vi "IO Channel Configuration.vi"() -> ()   [LabVIEW 2013]
panel:
  out "Sum Input Channel":string
  out "Division Input Channel":string
  out "Y Input Channel":string
  out "X Output Channnel":string
  out "X Input Channel":string
  out "Y Output Channel":string
  out "Z Output Channel":string
  out "Z Input Channel":string
  in  "OK Button":bool
  in  "Enable Y Output":bool=TRUE
  in  "Enable Y Input":bool=TRUE
  in  "Enable X Output":bool=TRUE
  in  "Enable X Input":bool=TRUE
  in  "Division Input Channel":tag
  in  "Sum Input Channel":tag
  in  "Z Output Channel":tag
  in  "Z Input Channel":tag
  in  "Y Output Channel":tag
  in  "Y Input Channel":tag
  in  "X Output Channel":tag
  in  "X Input Channel":tag
  # "Current Values:"
  # "Input/Ouput DAQmx Channel Selection:"
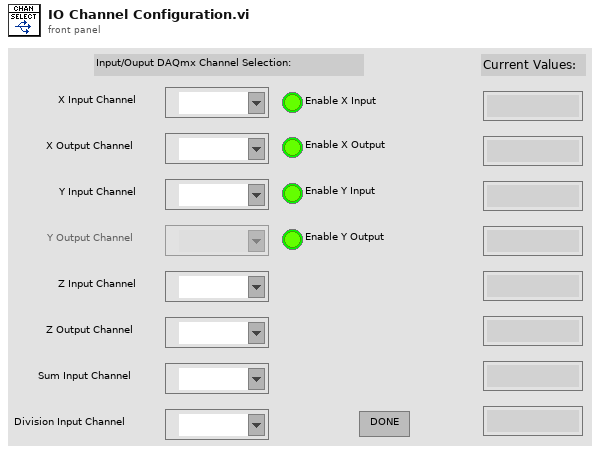
[diagram p1: front panel]
types:
  T1 = enum8{"Enabled", "Disabled", "Disabled and Grayed Out"}
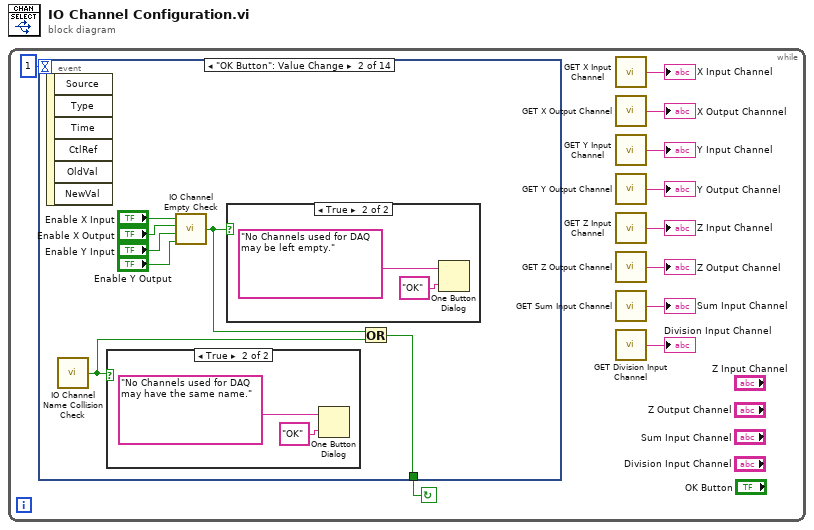
[diagram p0: block diagram]
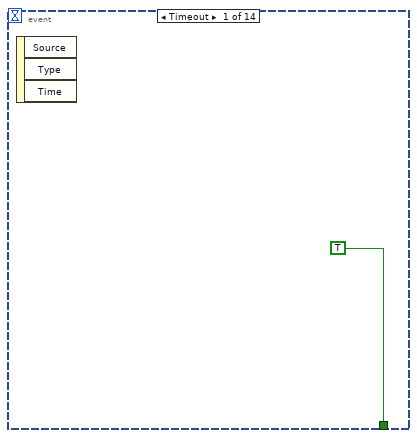
[diagram p2: hidden frame]
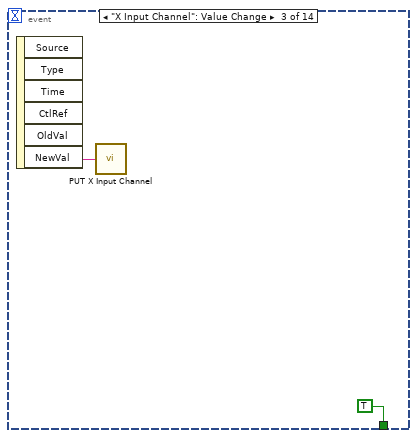
[diagram p5: hidden frame]
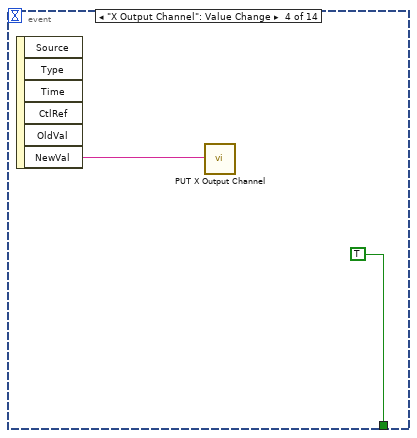
[diagram p6: hidden frame]
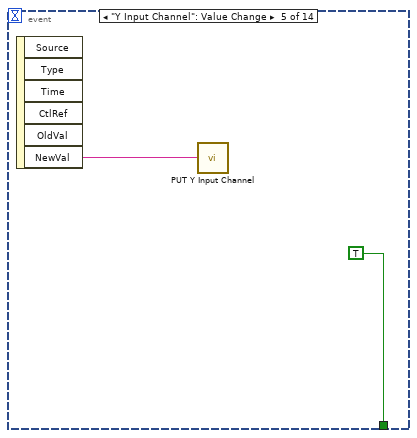
[diagram p7: hidden frame]
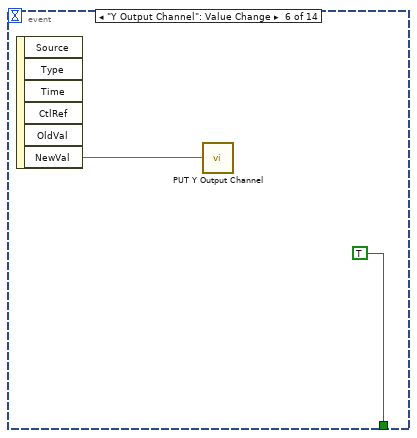
[diagram p8: hidden frame]
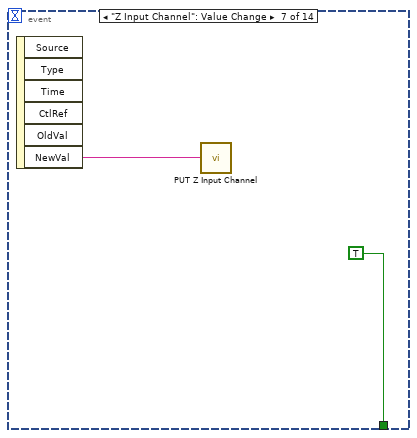
[diagram p9: hidden frame]
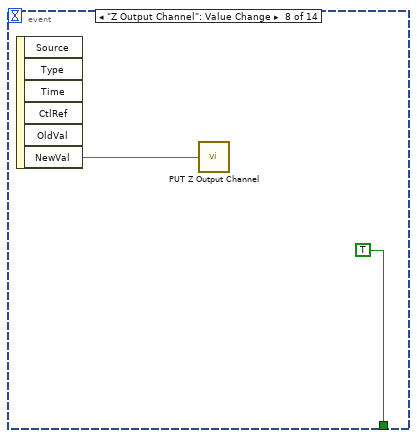
[diagram p10: hidden frame]
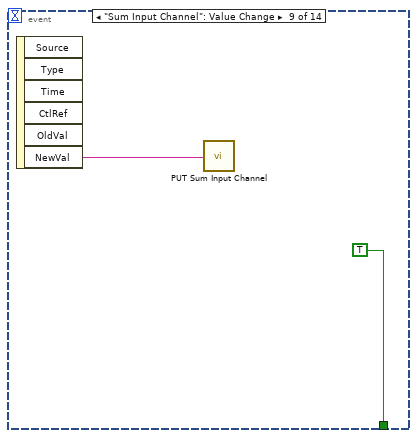
[diagram p11: hidden frame]
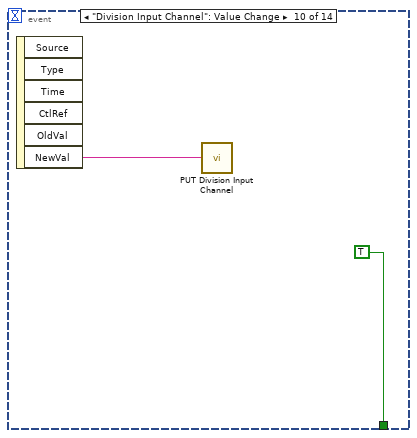
[diagram p12: hidden frame]
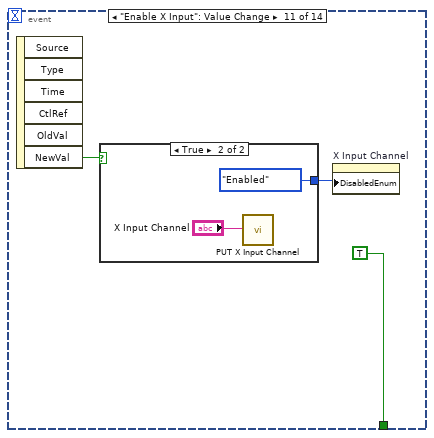
[diagram p13: hidden frame]
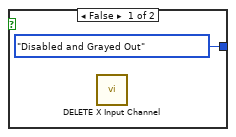
[diagram p14: hidden frame]
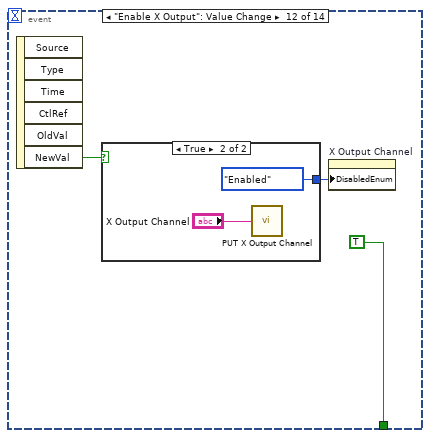
[diagram p15: hidden frame]
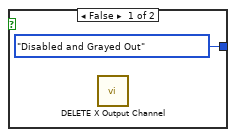
[diagram p16: hidden frame]
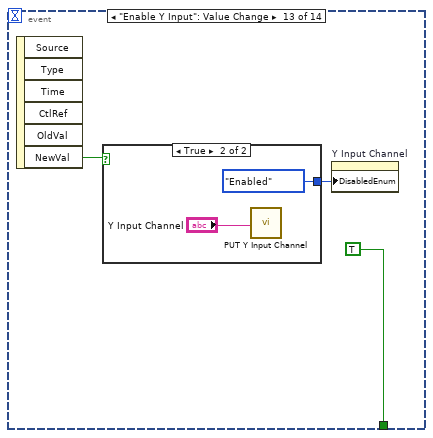
[diagram p17: hidden frame]
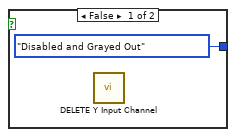
[diagram p18: hidden frame]
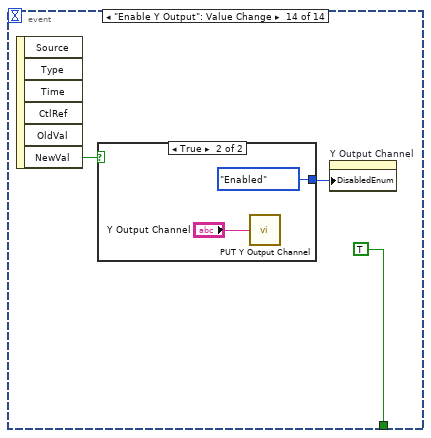
[diagram p19: hidden frame]
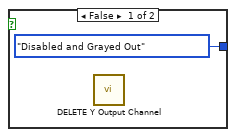
[diagram p20: hidden frame]
diagram:
  n1 = while {
    stop <- w10 continue-if-true
    n2 = event shown="[1] \"OK Button\": Value Change" {
      selector: _ -> [_ _ _ _ _ _ _ _ _ _ _ _ _ _]
      dyn-events: _ -> [_ _ _ _ _ _ _ _ _ _ _ _ _ _]
      timeout: 1 -> [_ _ _ _ _ _ _ _ _ _ _ _ _ _]
      tunnel: [TRUE w12 TRUE TRUE TRUE TRUE TRUE TRUE TRUE TRUE TRUE TRUE TRUE TRUE] -> w10
      event Timeout {
        n3 = event-data() -> ()  [unwired: 1 in, 3 out]
      }
      event "OK Button": Value Change {
        n4 = event-data() -> ()  [unwired: 1 in, 6 out]
        n5 = call "IO Channel Name Collision Check.vi"() -> ("Channel Names Collide"=w14:bool)
        n6 = case shown="True" w14 {
          frame False {
          }
          frame True {
            n7 = One Button Dialog(message="No Channels used for DAQ may have the same name.", button name ("OK")="OK") -> ()  [unwired: 1 out]
          }
        }
        n8 = call "IO Channel Empty Check.vi"("Enable Y Output"="Enable Y Output", "Enable Y Input"="Enable Y Input", "Enable X Output"="Enable X Output", "Enable X Input"="Enable X Input") -> ("Required Channels Empty"=w13:bool)
        n9 = case shown="True" w13 {
          frame False {
          }
          frame True {
            n10 = One Button Dialog(message="No Channels used for DAQ may be left empty.", button name ("OK")="OK") -> ()  [unwired: 1 out]
          }
        }
        n11 = Or(x=w13, y=w14) -> (x .or. y?=w12:bool)
      }
      event "X Input Channel": Value Change {
        n12 = event-data() -> ("NewVal"=w24:tag)  [unwired: 1 in, 5 out]
        n13 = call "PUT X Input Channel.vi"("X Input Channel"=w24) -> ()
      }
      event "X Output Channel": Value Change {
        n14 = event-data() -> ("NewVal"=w26:tag)  [unwired: 1 in, 5 out]
        n15 = call "PUT X Output Channel.vi"("X Output Channel"=w26) -> ()
      }
      event "Y Input Channel": Value Change {
        n16 = event-data() -> ("NewVal"=w28:tag)  [unwired: 1 in, 5 out]
        n17 = call "PUT Y Input Channel.vi"("Y Input Channel"=w28) -> ()
      }
      event "Y Output Channel": Value Change {
        n18 = event-data() -> ("NewVal"=w30:tag)  [unwired: 1 in, 5 out]
        n19 = call "PUT Y Output Channel.vi"("Y Output Channel"=w30) -> ()
      }
      event "Z Input Channel": Value Change {
        n20 = event-data() -> ("NewVal"=w32:tag)  [unwired: 1 in, 5 out]
        n21 = call "PUT Z Input Channel.vi"("Z Input Channel"=w32) -> ()
      }
      event "Z Output Channel": Value Change {
        n22 = event-data() -> ("NewVal"=w34:tag)  [unwired: 1 in, 5 out]
        n23 = call "PUT Z Output Channel.vi"("Z Output Channel"=w34) -> ()
      }
      event "Sum Input Channel": Value Change {
        n24 = event-data() -> ("NewVal"=w36:tag)  [unwired: 1 in, 5 out]
        n25 = call "PUT Sum Input Channel.vi"("Sum Input Channel"=w36) -> ()
      }
      event "Division Input Channel": Value Change {
        n26 = event-data() -> ("NewVal"=w38:tag)  [unwired: 1 in, 5 out]
        n27 = call "PUT Division Input Channel.vi"("Division Input Channel"=w38) -> ()
      }
      event "Enable X Input": Value Change {
        n28 = event-data() -> ("NewVal"=w41:bool)  [unwired: 1 in, 5 out]
        n29 = case shown="True" w41 {
          tunnel: [T1."Disabled and Grayed Out" ("Disabled") T1."Enabled" ("Disabled")] -> w40
          frame False {
            n30 = call "DELETE X Input Channel.vi"() -> ()  [unwired: 1 in]
          }
          frame True {
            n31 = call "PUT X Input Channel.vi"("X Input Channel"="X Input Channel") -> ()
          }
        }
        n32 = property on="X Input Channel" class="DAQmxName"("DisabledEnum"=w40) -> ()  [unwired: 2 in, 2 out]
      }
      event "Enable X Output": Value Change {
        n33 = event-data() -> ("NewVal"=w47:bool)  [unwired: 1 in, 5 out]
        n34 = case shown="True" w47 {
          tunnel: [T1."Disabled and Grayed Out" ("Disabled") T1."Enabled" ("Disabled")] -> w46
          frame False {
            n35 = call "DELETE X Output Channel.vi"() -> ()  [unwired: 1 in]
          }
          frame True {
            n36 = call "PUT X Output Channel.vi"("X Output Channel"="X Output Channel") -> ()
          }
        }
        n37 = property on="X Output Channel" class="DAQmxName"("DisabledEnum"=w46) -> ()  [unwired: 2 in, 2 out]
      }
      event "Enable Y Input": Value Change {
        n38 = event-data() -> ("NewVal"=w53:bool)  [unwired: 1 in, 5 out]
        n39 = case shown="True" w53 {
          tunnel: [T1."Disabled and Grayed Out" ("Disabled") T1."Enabled" ("Disabled")] -> w52
          frame False {
            n40 = call "DELETE Y Input Channel.vi"() -> ()  [unwired: 1 in]
          }
          frame True {
            n41 = call "PUT Y Input Channel.vi"("Y Input Channel"="Y Input Channel") -> ()
          }
        }
        n42 = property on="Y Input Channel" class="DAQmxName"("DisabledEnum"=w52) -> ()  [unwired: 2 in, 2 out]
      }
      event "Enable Y Output": Value Change {
        n43 = event-data() -> ("NewVal"=w59:bool)  [unwired: 1 in, 5 out]
        n44 = case shown="True" w59 {
          tunnel: [T1."Disabled and Grayed Out" ("Disabled") T1."Enabled" ("Disabled")] -> w57
          frame False {
            n45 = call "DELETE Y Output Channel.vi"() -> ()  [unwired: 1 in]
          }
          frame True {
            n46 = call "PUT Y Output Channel.vi"("Y Output Channel"="Y Output Channel") -> ()
          }
        }
        n47 = property on="Y Output Channel" class="DAQmxName"("DisabledEnum"=w57) -> ()  [unwired: 2 in, 2 out]
      }
    }
    n48 = call "GET X Input Channel.vi"() -> ("X Input Channel"=→"X Input Channel":string)
    n49 = call "GET X Output Channel.vi"() -> ("X Output Channel"=→"X Output Channnel":string)
    n50 = call "GET Y Input Channel.vi"() -> ("Y Input Channel"=→"Y Input Channel":string)
    n51 = call "GET Y Output Channel.vi"() -> ("Y Output Channel"=→"Y Output Channel":string)
    n52 = call "GET Z Input Channel.vi"() -> ("Z Input Channel"=→"Z Input Channel":string)
    n53 = call "GET Z Output Channel.vi"() -> ("Z Output Channel"=→"Z Output Channel":string)
    n54 = call "GET Sum Input Channel.vi"() -> ("Sum Input Channel"=→"Sum Input Channel":string)
    n55 = call "GET Division Input Channel.vi"() -> ("Division Input Channel"=→"Division Input Channel":string)
  }
